vi "ParseStepIndex.vi"(8 "error in (no error)":errorcluster, 11 "Data":variant) -> (0 "error out":errorcluster, 3 "StepIndex":T1)   [LabVIEW 2016, in "SeqProcessor.lvlib"]
uses:
  SeqProcessor.lvlib
  controls/StepIndex.ctl
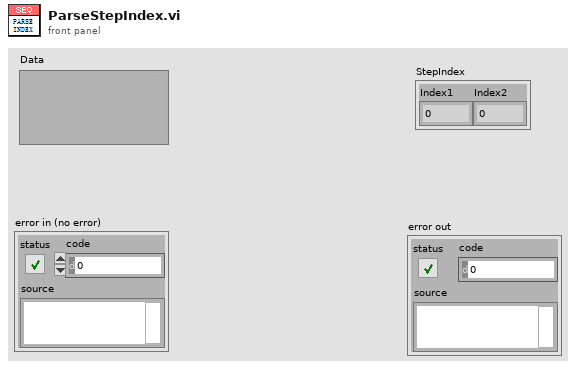
[diagram p1: front panel]
types:
  T1 = typedef "SeqProcessor.lvlib/StepIndex.ctl" = cluster{"Index1":u32, "Index2":u32}
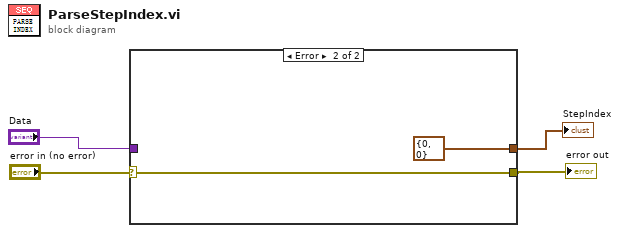
[diagram p0: block diagram]
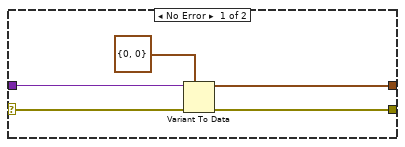
[diagram p2: hidden frame]
diagram:
  n1 = case shown="Error" "error in (no error)" {
    selector: "error in (no error)" -> [w6 w11]
    tunnel: "Data" -> [w9 _]
    tunnel: [w7 T1 {"Index1"=0, "Index2"=0} ("Index")] -> w3
    tunnel: [w5 w11] -> w1
    frame No Error {
      n2 = Variant To Data(error in=w6, type=T1 {"Index1"=0, "Index2"=0} ("Index"), Variant=w9) -> (data=w7:T1, error out=w5:errorcluster)
    }
    frame Error {
    }
  }
  "error out" <- w1
  "StepIndex" <- w3
